vi "lat_lon to string.vi"(9 "lat/lon":u16(ring) items=["Latitude", "Longitude", "Variation"], 10 "composite value":dbl) -> (2 "NMEA string for lat/lon":string)   [LabVIEW 2017, in "NMEA API.lvlib"]
uses:
  <vilib>/robotics/Protocols/NMEA/NMEA API.lvlib
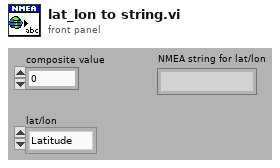
[diagram p1: front panel]
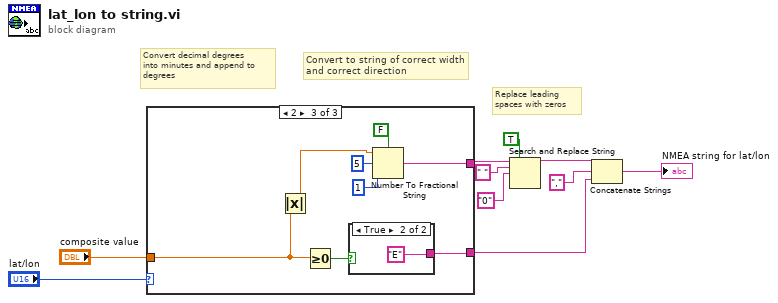
[diagram p0: block diagram]
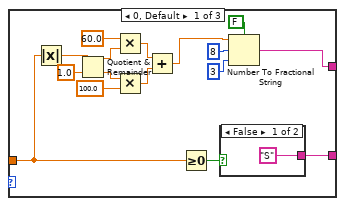
[diagram p2: hidden frame]
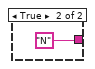
[diagram p3: hidden frame]
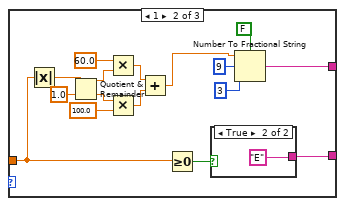
[diagram p4: hidden frame]
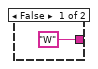
[diagram p5: hidden frame]
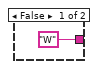
[diagram p6: hidden frame]
diagram:
  # "Replace leading\nspaces with zeros"
  # "Convert to string of correct width\nand correct direction"
  # "Convert decimal degrees\ninto minutes and append to\ndegrees"
  n1 = case shown="2" "lat/lon" {
    tunnel: "composite value" -> [w13 w31 w49]
    tunnel: [w25 w43 w53] -> w8
    tunnel: [w22 w40 w50] -> w5
    frame 0, Default {
      n2 = Absolute Value(x=w13) -> (abs(x)=w14:dbl)
      n3 = Quotient & Remainder(x=w14, y=1.0) -> (x-y*floor(x/y)=w18:dbl, floor(x/y)=w20:dbl)
      n4 = Multiply(x=60.0, y=w18) -> (x*y=w15:dbl)
      n5 = Multiply(x=w20, y=100.0) -> (x*y=w16:dbl)
      n6 = Add(x=w15, y=w16) -> (x+y=w12:dbl)
      n7 = Greater Or Equal To 0?(x=w13) -> (x >= 0?=w26:bool)
      n8 = case shown="False" w26 {
        tunnel: ["S" "N"] -> w25
        frame False {
        }
        frame True {
        }
      }
      n9 = Number To Fractional String(use system decimal point (T)=FALSE, number=w12, width (-)=i16 8, precision (6)=i16 3) -> (F-format string=w22:string)
    }
    frame 1 {
      n10 = Absolute Value(x=w31) -> (abs(x)=w39:dbl)
      n11 = Quotient & Remainder(x=w39, y=1.0) -> (x-y*floor(x/y)=w35:dbl, floor(x/y)=w33:dbl)
      n12 = Multiply(x=60.0, y=w35) -> (x*y=w38:dbl)
      n13 = Multiply(x=w33, y=100.0) -> (x*y=w37:dbl)
      n14 = Add(x=w38, y=w37) -> (x+y=w30:dbl)
      n15 = Greater Or Equal To 0?(x=w31) -> (x >= 0?=w44:bool)
      n16 = case shown="True" w44 {
        tunnel: ["W" "E"] -> w43
        frame False {
        }
        frame True {
        }
      }
      n17 = Number To Fractional String(use system decimal point (T)=FALSE, number=w30, width (-)=i16 9, precision (6)=i16 3) -> (F-format string=w40:string)
    }
    frame 2 {
      n18 = Absolute Value(x=w49) -> (abs(x)=w48:dbl)
      n19 = Greater Or Equal To 0?(x=w49) -> (x >= 0?=w54:bool)
      n20 = case shown="True" w54 {
        tunnel: ["W" "E"] -> w53
        frame False {
        }
        frame True {
        }
      }
      n21 = Number To Fractional String(use system decimal point (T)=FALSE, number=w48, width (-)=i16 5, precision (6)=i16 1) -> (F-format string=w50:string)
    }
  }
  n22 = Search and Replace String(replace all?=TRUE ("replace all? (F)"), input string=w5, search string=" ", replace string="0" ("replace string (\"\")")) -> (result string=w2:string)  [unwired: 1 in, 6 out]
  n23 = Concatenate Strings(w2, "," ("string"), w8) -> (→"NMEA string for lat/lon":string)
